vi "Flatten Variant to JSON.vi"(6 "pretty print? (F)":bool, 7 "enable LabVIEW extensions? (T)":bool=TRUE, 8 "error in (no error)":errorcluster, 11 "JSON Value in":variant) -> (0 "error out":errorcluster, 3 "String":string)   [LabVIEW 2017, in "Advanced Variant Tools.lvlib"]
uses:
  Advanced Variant Tools.lvlib
  JSON Support.lvlib
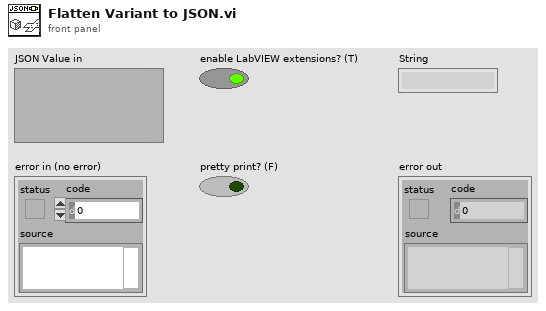
[diagram p1: front panel]
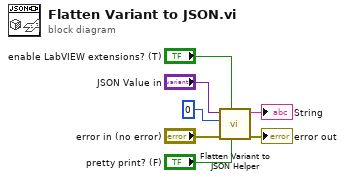
[diagram p0: block diagram]
diagram:
  n1 = call "Flatten Variant to JSON Helper.vi"("pretty print? (T)"="pretty print? (F)", "enable LabVIEW extensions? (T)"="enable LabVIEW extensions? (T)", "error in (no error)"="error in (no error)", "indent"=0, "JSON Value in"="JSON Value in") -> ("error out"=→"error out":errorcluster, "String"=→"String":string)  [unwired: 5 in]
